vi "Test read variables.vi"() -> ()   [LabVIEW 2015]
uses:
  <resource>/objmgr/ni.var.rc
  <vilib>/Utility/VariantDataType/VariantType.lvlib
panel:
  out "Boolean":bool[](array[boolean])
  out "Double":dbl[](array[numeric])
  in  "Boolean":bool
  in  "Shared Variable Library Name":string="Shared Variable Test Library cRIO"
  in  "IP Address":string="10.118.8.160"
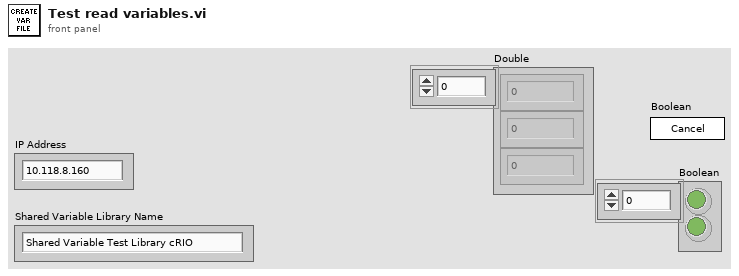
[diagram p1: front panel]
types:
  T1 = typedef "VariantType.lvlib/Type.ctl" = enum8{"Invalid Type", "Void", "I8", "I16", "I32", "I64", "U8", "U16", "U32", "U64", "Single Float", "Double Float", "Extended Float", "Single Complex", "Double Complex", "Extended Complex", "Enum U8", "Enum U16", "Enum U32", "Enum U64", "Single Float With Unit", "Double Float With Unit", "Extended Float With Unit", "Single Complex with Unit", "Double Complex with Unit", "Extended Complex with Unit", "Boolean", "String", "Path", "Picture", "Tag", "Array", "Cluster", "Variant", "LV Variant", "Waveform", "Timestamp", "Digital Waveform", "Digital Data", "ExpressData", "Refnum", "External Data", "VI", "Poly VI", "LabVIEW Class Instance", "Fixed Point"}
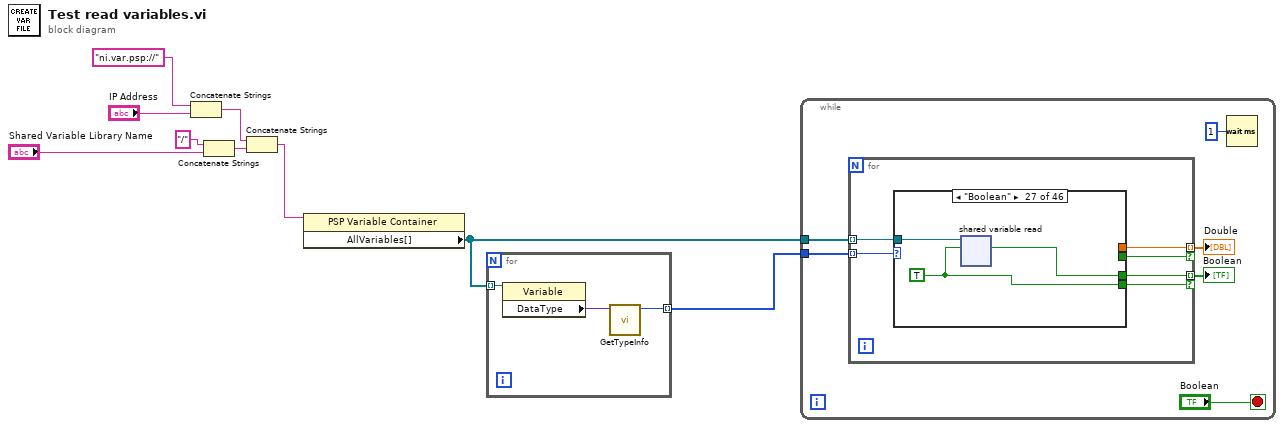
[diagram p0: block diagram]
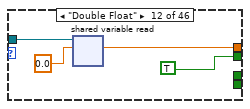
[diagram p13: hidden frame]
diagram:
  n1 = Concatenate Strings("ni.var.psp://" ("PSP URL"), "IP Address") -> (w4:string)
  n2 = Concatenate Strings("/" ("string"), "Shared Variable Library Name") -> (w5:string)
  n3 = Concatenate Strings(w4, w5) -> (w3:string)
  n4 = property class="PSP Variable Container"(reference=w3) -> ("AllVariables[]"=w2:refnum<k21>[])  [unwired: 1 in, 2 out]
  n5 = for {
    tunnel: w2 -> [w11] mode=indexing
    tunnel: [w10] -> w1 mode=indexing
    n6 = property class="Variable"(reference=w11) -> ("DataType"=w12:variant)  [unwired: 1 in, 2 out]
    n7 = call <vilib>:"GetTypeInfo.vi"("Variant"=w12) -> ("Type Enum"=w10:T1)  [unwired: 6 in, 4 out]
  }
  n8 = while {
    tunnel: w2 -> [w18]
    tunnel: w1 -> [w15]
    stop <- "Boolean" stop-if-true
    n9 = for {
      tunnel: w18 -> [w24] mode=indexing
      tunnel: w15 -> [w23] mode=indexing
      tunnel: [w22] -> w14 mode=indexing if=w21
      tunnel: [w20] -> w13 mode=indexing if=w19
      n10 = case shown="\"Boolean\"" w23 {
        tunnel: w24 -> [_ _ _ _ _ _ _ _ _ _ _ w28 _ _ _ _ _ _ _ _ _ _ _ _ _ _ w31 _ _ _ _ _ _ _ _ _ _ _ _ _ _ _ _ _ _ _]
        tunnel: [_ _ _ _ _ _ _ _ _ _ _ w26 _ _ _ _ _ _ _ _ _ _ _ _ _ _ _ _ _ _ _ _ _ _ _ _ _ _ _ _ _ _ _ _ _ _] -> w22
        tunnel: [_ _ _ _ _ _ _ _ _ _ _ TRUE _ _ _ _ _ _ _ _ _ _ _ _ _ _ _ _ _ _ _ _ _ _ _ _ _ _ _ _ _ _ _ _ _ _] -> w21
        tunnel: [_ _ _ _ _ _ _ _ _ _ _ _ _ _ _ _ _ _ _ _ _ _ _ _ _ _ w30 _ _ _ _ _ _ _ _ _ _ _ _ _ _ _ _ _ _ _] -> w20
        tunnel: [_ _ _ _ _ _ _ _ _ _ _ _ _ _ _ _ _ _ _ _ _ _ _ _ _ _ w29 _ _ _ _ _ _ _ _ _ _ _ _ _ _ _ _ _ _ _] -> w19
        frame "Invalid Type", Default {
        }
        frame "Void" {
        }
        frame "I8" {
        }
        frame "I16" {
        }
        frame "I32" {
        }
        frame "I64" {
        }
        frame "U8" {
        }
        frame "U16" {
        }
        frame "U32" {
        }
        frame "U64" {
        }
        frame "Single Float" {
        }
        frame "Double Float" {
          n11 = shared-variable-read(w28, 0.0) -> (w26:dbl)  [unwired: 1 in, 3 out]
        }
        frame "Extended Float" {
        }
        frame "Single Complex" {
        }
        frame "Double Complex" {
        }
        frame "Extended Complex" {
        }
        frame "Enum U8" {
        }
        frame "Enum U16" {
        }
        frame "Enum U32" {
        }
        frame "Enum U64" {
        }
        frame "Single Float With Unit" {
        }
        frame "Double Float With Unit" {
        }
        frame "Extended Float With Unit" {
        }
        frame "Single Complex with Unit" {
        }
        frame "Double Complex with Unit" {
        }
        frame "Extended Complex with Unit" {
        }
        frame "Boolean" {
          w29 = TRUE
          n12 = shared-variable-read(w31, w29) -> (w30:bool)  [unwired: 1 in, 3 out]
        }
        frame "String" {
        }
        frame "Path" {
        }
        frame "Picture" {
        }
        frame "Tag" {
        }
        frame "Array" {
        }
        frame "Cluster" {
        }
        frame "Variant" {
        }
        frame "LV Variant" {
        }
        frame "Waveform" {
        }
        frame "Timestamp" {
        }
        frame "Digital Waveform" {
        }
        frame "Digital Data" {
        }
        frame "ExpressData" {
        }
        frame "Refnum" {
        }
        frame "External Data" {
        }
        frame "VI" {
        }
        frame "Poly VI" {
        }
        frame "LabVIEW Class Instance" {
        }
        frame "Fixed Point" {
        }
      }
    }
    "Double" <- w14
    "Boolean" <- w13
    n13 = Wait (ms)(milliseconds to wait=u32 1) -> ()  [unwired: 1 out]
  }
